vi "Write receive on port.vi"(8 "error in":errorcluster, 10 "receive on port":u16=61555, 11 "TEC configuration in":refnum<class "TEC configuration.lvclass">) -> (0 "error out":errorcluster, 3 "TEC configuration out":refnum<class "TEC configuration.lvclass">)   [LabVIEW 2013, in "TEC configuration.lvclass"]
uses:
  TEC configuration.lvclass
  TEC configuration.lvclass/TEC configuration.ctl
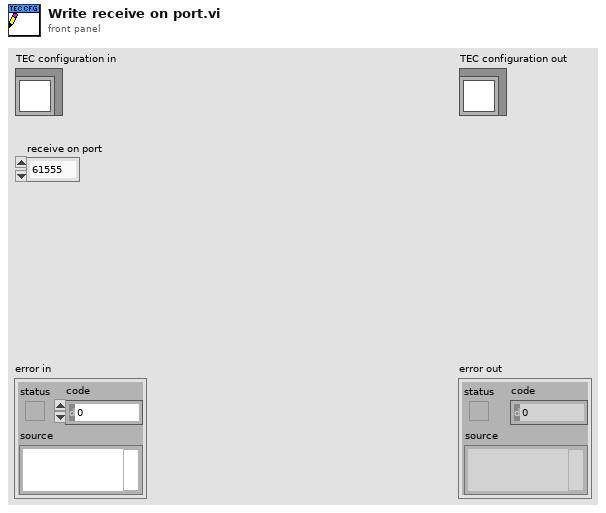
[diagram p1: front panel]
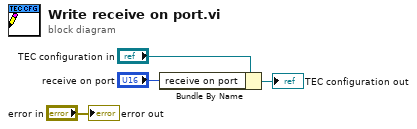
[diagram p0: block diagram]
diagram:
  n1 = Bundle By Name(cluster="TEC configuration in", "receive on port"="receive on port") -> (→"TEC configuration out":refnum<class "TEC configuration.lvclass">)
  "error out" <- "error in"
